vi "Parse API JSON Response.vi"(8 "error in":errorcluster, 11 "API Response":string) -> (0 "error out":errorcluster, 3 "Results":T1(array[cluster]))   [LabVIEW 2025, in "Geocoding Actor.lvlib" / "Geocoding.lvclass"]
uses:
  Geocoding.lvclass
  Geocoding.lvclass/Geocoding.ctl
  <vilib>/addons/_JKI.lib/Serialization/JSON/JKI JSON Serialization.lvlib
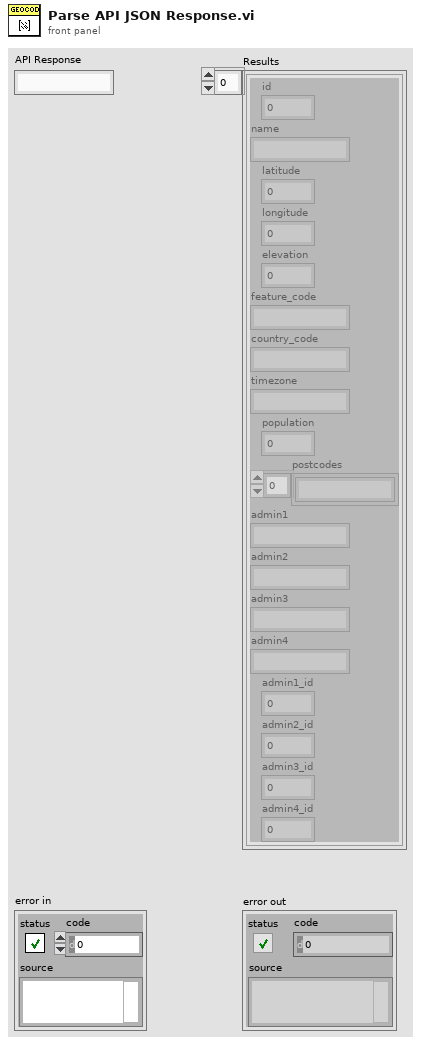
[diagram p1: front panel]
types:
  T1 = cluster{"id":i32, "name":string, "latitude":dbl, "longitude":dbl, "elevation":dbl, "feature_code":string, "country_code":string, "timezone":string, "population":i32, "postcodes":string[], "admin1":string, "admin2":string, "admin3":string, "admin4":string, "admin1_id":i32, "admin2_id":i32, "admin3_id":i32, "admin4_id":i32}[]
  T2 = cluster{"results":cluster{"id":i32, "name":string, "latitude":dbl, "longitude":dbl, "elevation":dbl, "feature_code":string, "country_code":string, "timezone":string, "population":i32, "postcodes":string[], "admin1":string, "admin2":string, "admin3":string, "admin4":string, "admin1_id":i32, "admin2_id":i32, "admin3_id":i32, "admin4_id":i32}[], "generationtime_ms":dbl}
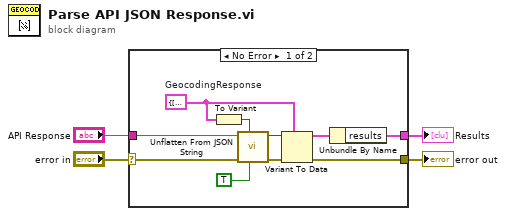
[diagram p0: block diagram]
diagram:
  n1 = case shown="No Error" "error in" {
    selector: "error in" -> [w8 w15]
    tunnel: "API Response" -> [w9 _]
    tunnel: [w7 w15] -> w2
    tunnel: [w5 _] -> w1
    frame No Error {
      w10 = T2 {"results"=[], "generationtime_ms"=0.0}  # GeocodingResponse
      n2 = To Variant(anything=w10) -> (Variant=w11:variant)
      n3 = call <vilib>:"Unflatten From JSON String.vi"("Nulls as Defaults (F)"=TRUE, "Type and Defaults"=w11, "error in"=w8, "JSON String"=w9) -> ("error out"=w12:errorcluster, "Variant"=w13:variant)  [unwired: 6 in]
      n4 = Variant To Data(error in=w12, type=w10, Variant=w13) -> (data=w6:T2, error out=w7:errorcluster)
      n5 = Unbundle By Name(w6) -> ("results"=w5:T1)
    }
    frame Error {
    }
  }
  "error out" <- w2
  "Results" <- w1
